vi "Get PCL Decimation.vi"(8 "error in (no error)":errorcluster, 11 "instrument addon refnum in":T1=18446744073709551615 format="%.0x") -> (0 "error out":errorcluster, 2 "PCL decimation":u32, 3 "instrument addon refnum out":T1=18446744073709551615 format="%.0x")   [LabVIEW 2019, in "Scripting API.lvlib"]
uses:
  Scripting API.lvlib
  <vilib>/NI VeriStand/Custom Device API/Custom Device Item Ref.ctl
  <vilib>/NI VeriStand/Custom Device API/Custom Device API.lvlib
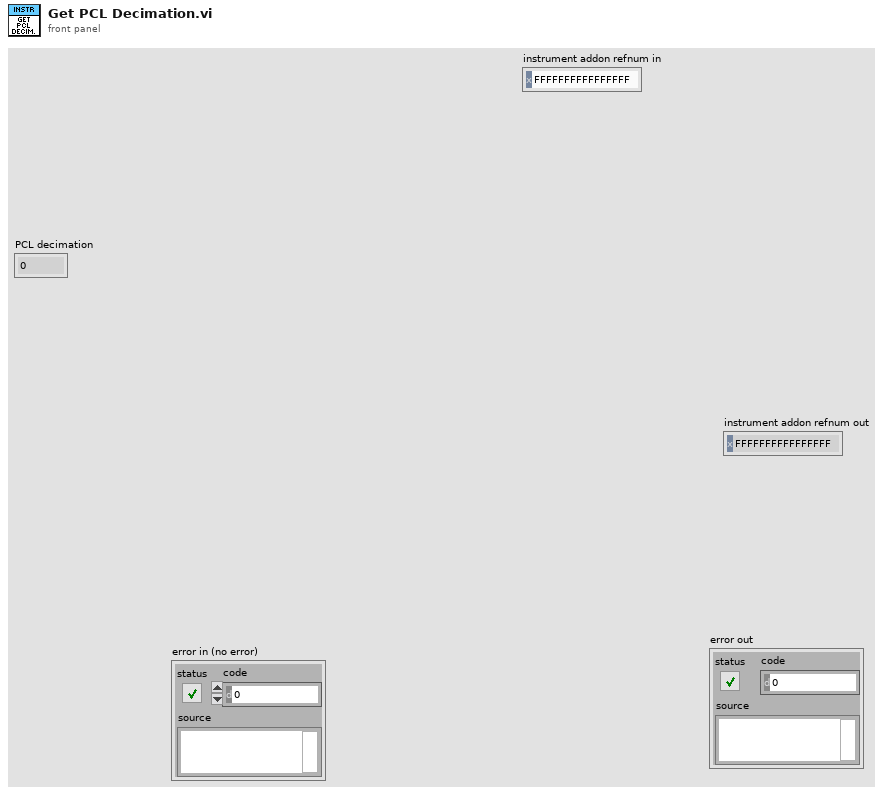
[diagram p1: front panel]
types:
  T1 = typedef "Custom Device API.lvlib/Custom Device Item Ref.ctl" = u64
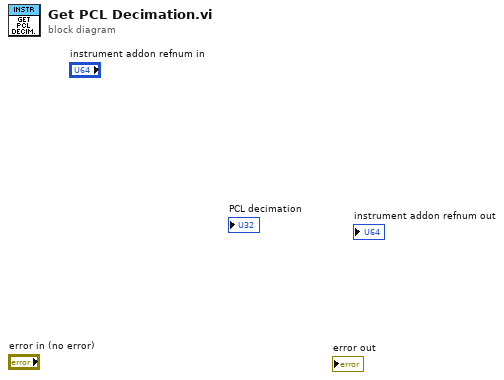
[diagram p0: block diagram]
diagram:
